vi "MotionTracker2DCorr.vi"(4 "Ref frame for 2S":i32=1, 6 "Cursor.Cursor Position":T1, 7 "#x lines":i32, 9 "#y rf":i32, 10 "RF In":sgl[][][](array[numeric]), 11 "2D threshold":sgl=19.0) -> (1 "Mean axial Disp":dbl[](graph), 2 "2D corr":dbl[][](graph), 3 "Peak tracker":dbl[][](array[numeric]))   [LabVIEW 2022 SP3]
uses:
  <vilib>/Utility/miscctls.llb/LVPointDoubleTypeDef.ctl
  <vilib>/Analysis/2dsp.llb/2D Cross Correlation (DBL).vi
  <vilib>/Analysis/baseanly.llb/Mean (DBL).vi
  <vilib>/Analysis/NI_AALBase.lvlib
  <vilib>/Analysis/NI_AALPro.lvlib
panel:
  out "rawx pk":dbl[](graph)
  out "abs distance":dbl[](graph)
  out "raw axial pk":dbl[](graph)
  out "mean X displacment":dbl[](graph)
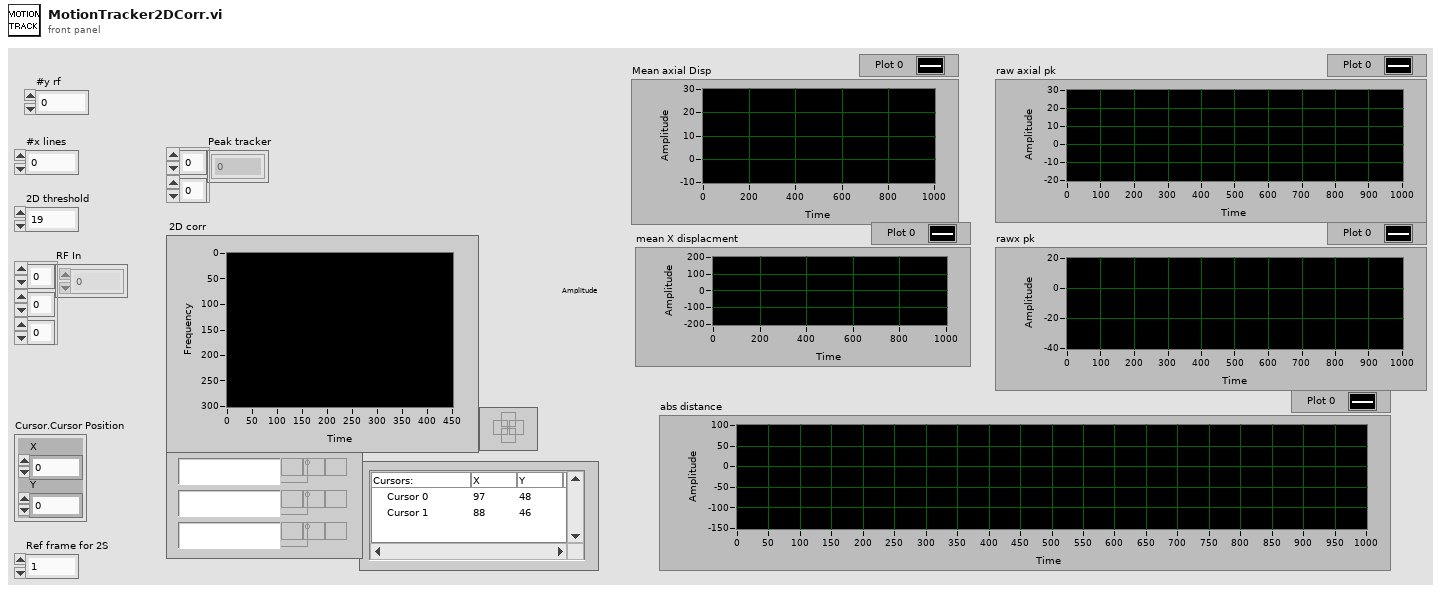
[diagram p1: front panel]
types:
  T1 = typedef "LVPointDoubleTypeDef.ctl" = cluster{"X":dbl, "Y":dbl}
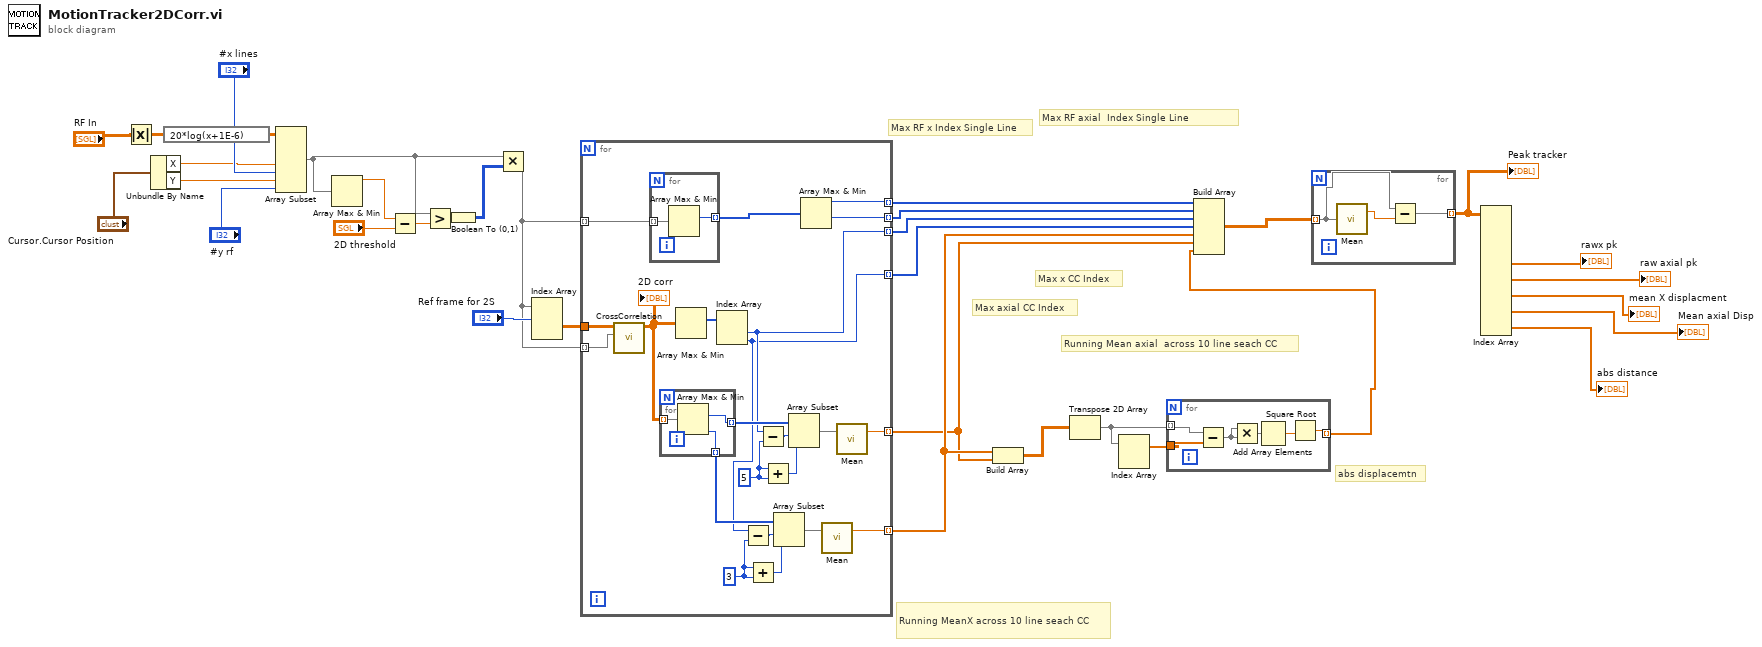
[diagram p0: block diagram]
diagram:
  # "Max x CC Index"
  # "Max RF axial  Index Single Line"
  # "Running MeanX across 10 line seach CC"
  # "Running Mean axial  across 10 line seach CC"
  # "Max axial CC Index"
  # "abs displacemtn"
  # "Max RF x Index Single Line"
  n1 = Absolute Value(x="RF In") -> (abs(x)=w3:sgl[][][])
  n2 = Unbundle By Name("Cursor.Cursor Position") -> ("X"=w23:dbl, "Y"=w32:dbl)
  n3 = expression code="20*log(x+1E-6)"(w3) -> (w1:sgl[][][])
  n4 = Array Subset(array=w1, index (dim 1)=w23, length (dim 1)="#x lines", index (dim 2)=w32, length (dim 2)="#y rf") -> (w21:sgl[][][])  [unwired: 2 in]
  n5 = Array Max & Min(array=w21) -> (max value=w27:sgl)  [unwired: 3 out]
  n6 = Subtract(x=w27, y="2D threshold") -> (x-y=w29:sgl)
  n7 = Greater?(x=w21, y=w29) -> (0:w30:bool[][][])
  n8 = Boolean To (0,1)(Boolean=w30) -> (0, 1=w31:i16[][][])
  n9 = Multiply(x=w21, y=w31) -> (x*y=w20:sgl[][][])
  n10 = Index Array(array=w20, index (dim 0)="Ref frame for 2S") -> (element=w33:sgl[][])  [unwired: 2 in]
  n11 = for {
    tunnel: w20 -> [w35] mode=indexing
    tunnel: [w55] -> w22 mode=indexing
    tunnel: w33 -> [w54]
    tunnel: [w36] -> w15 mode=indexing
    tunnel: w20 -> [w53] mode=indexing
    tunnel: [w47] -> w9 mode=indexing
    tunnel: [w39] -> w10 mode=indexing
    tunnel: [w38] -> w16 mode=indexing
    tunnel: [w37] -> w14 mode=indexing
    w43 = 3 ("y")
    w50 = 5 ("y")
    n12 = call-poly <vilib>:"CrossCorrelation.vi"("Y"=w53, "X"=w54) -> ("Rxy"=w46:dbl[][])  [unwired: 8 in, 1 out]
    "2D corr" <- w46
    n13 = for {
      tunnel: w35 -> [w61] mode=indexing
      tunnel: [w60] -> w56 mode=indexing
      n14 = Array Max & Min(array=w61) -> (max index (indices)=w60:i32)  [unwired: 3 out]
    }
    n15 = for {
      tunnel: w46 -> [w59] mode=indexing
      tunnel: [w58] -> w52 mode=indexing
      tunnel: [w57] -> w40 mode=indexing
      n16 = Array Max & Min(array=w59) -> (max index (indices)=w58:i32, min index (indices)=w57:i32)  [unwired: 2 out]
    }
    n17 = Array Max & Min(array=w46) -> (max index (indices)=w45:i32[])  [unwired: 3 out]
    n18 = Index Array(array=w45) -> (element #1=w37:i32, element #2=w36:i32)  [unwired: 2 in]
    n19 = Subtract(x=w36, y=w43) -> (x-y=w44:i32)
    n20 = Add(x=w43, y=w43) -> (x+y=w42:i32)
    n21 = Subtract(x=w37, y=w50) -> (x-y=w51:i32)
    n22 = Add(x=w50, y=w50) -> (x+y=w49:i32)
    n23 = Array Subset(array=w40, index=w44, length=w42) -> (w41:i32[])
    n24 = Array Subset(array=w52, index=w51, length=w49) -> (w48:i32[])
    n25 = Array Max & Min(array=w56) -> (max value=w55:i32, min value=w38:i32)  [unwired: 2 out]
    n26 = call-poly <vilib>:"Mean.vi"("X"=w41) -> ("mean"=w39:dbl)  [unwired: 1 out]
    n27 = call-poly <vilib>:"Mean.vi"("X"=w48) -> ("mean"=w47:dbl)  [unwired: 1 out]
  }
  n28 = Build Array(w10, w9) -> (w18:dbl[][])
  n29 = Transpose 2D Array(2D array=w18) -> (transposed array=w17:dbl[][])
  n30 = Index Array(array=w17) -> (element=w19:dbl[])  [unwired: 2 in]
  n31 = for {
    tunnel: w17 -> [w67] mode=indexing
    tunnel: w19 -> [w66]
    tunnel: [w62] -> w5 mode=indexing
    n32 = Subtract(x=w67, y=w66) -> (x-y=w65:dbl[])
    n33 = Multiply(x=w65, y=w65) -> (x*y=w64:dbl[])
    n34 = Add Array Elements(numeric array=w64) -> (sum=w63:dbl)
    n35 = Square Root(x=w63) -> (sqrt(x)=w62:dbl)
  }
  n36 = Build Array(w22, w16, w14, w15, w10, w9, w5) -> (w13:dbl[][])
  n37 = for {
    tunnel: w13 -> [w68] mode=indexing
    tunnel: [w69] -> w6 mode=indexing
    n38 = call-poly <vilib>:"Mean.vi"("X"=w68) -> ("mean"=w70:dbl)  [unwired: 1 out]
    n39 = Subtract(x=w68, y=w70) -> (x-y=w69:dbl[])
  }
  "Peak tracker" <- w6
  n40 = Index Array(array=w6) -> (element #3=→"rawx pk":dbl[], element #4=→"raw axial pk":dbl[], element #5=→"mean X displacment":dbl[], element #6=→"Mean axial Disp":dbl[], element #7=→"abs distance":dbl[])  [unwired: 14 in, 2 out]
